vi "repaint.vi"(0 "reference":refnum<class "Graphics.lvclass">, 5 "error in (no error)":errorcluster) -> (14 "reference out":refnum<class "Graphics.lvclass">, 19 "error out":errorcluster)   [LabVIEW 2016, in "Graphics.lvclass"]
uses:
  <resource>/Framework/Providers/Open_GDS/UML/Graphics_class/Graphics.lvclass
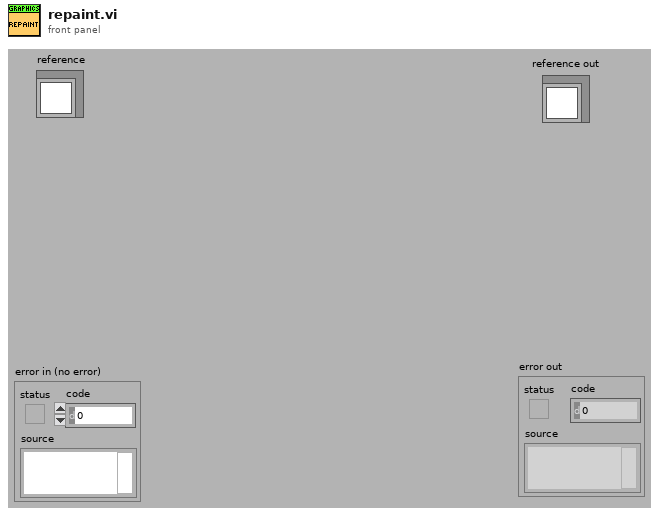
[diagram p1: front panel]
types:
  T1 = typedef "Graphics.lvclass/ObjectAttributes.ctl" = cluster{"drawColor":u32, "backgroundColor":u32, "font":T2, "fontType":T3, "picture":picture, "stroke":T4, "scaleX":dbl, "scaleY":dbl, "screenRef":refnum<vi>, "offsetX":dbl, "offsetY":dbl}
  T2 = typedef "Graphics.lvclass/FontType.ctl" = cluster{"Font Name:":string, "Size":i16, "Strikeout?":bool, "Italic?":bool, "Underline?":bool, "Outline?":bool, "Shadow?":bool, "Bold?":bool}
  T3 = typedef "Graphics.lvclass/LvFontType.ctl" = enum16{"User-specified Font", "Application Font", "System Font", "Dialog Font"}
  T4 = typedef "Graphics.lvclass/StrokeType.ctl" = enum16{"USE_DEFAULT", "SOLID", "DOTTED"}
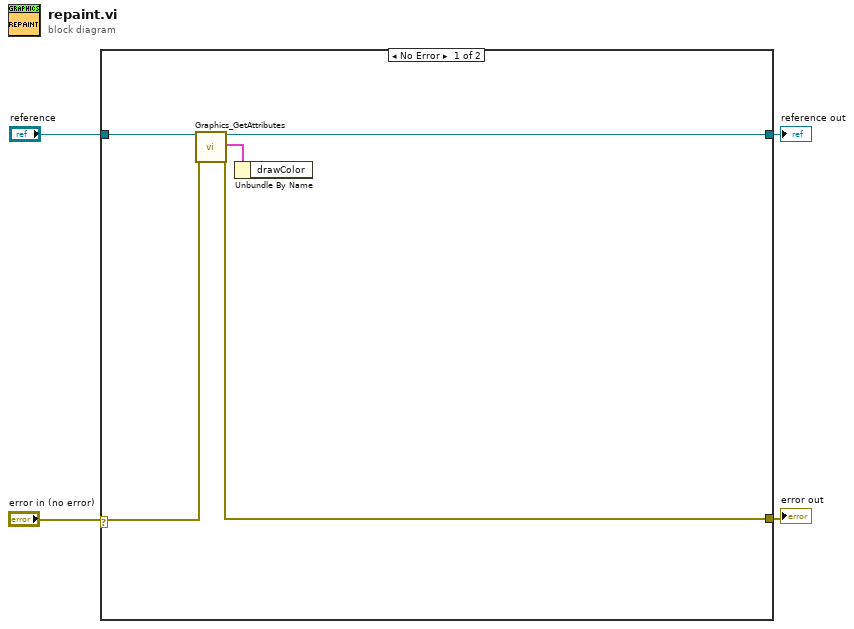
[diagram p0: block diagram]
diagram:
  n1 = case shown="No Error" "error in (no error)" {
    selector: "error in (no error)" -> [w6 w10]
    tunnel: "reference" -> [w9 w11]
    tunnel: [w8 w10] -> w3
    tunnel: [w7 w11] -> w2
    frame No Error {
      n2 = call <resource>:"Graphics_GetAttributes.vi"("reference in"=w9, "error in (no error)"=w6) -> ("reference out"=w7:refnum<class "Graphics.lvclass">, "Data"=w5:T1, "error out"=w8:errorcluster)  [unwired: 1 in, 14 out]
      n3 = Unbundle By Name(w5) -> ()  [unwired: 1 out]
    }
    frame Error {
    }
  }
  "reference out" <- w2
  "error out" <- w3
